vi "Find Previous File.vi"(7 "Baseline Directory":path, 8 "error in":errorcluster, 10 "Relative Path":string, 11 "Response String":string) -> (0 "error out":errorcluster, 3 "Previous Name":path)   [LabVIEW 2020, in "Peer Review.lvclass"]
uses:
  Peer Review.lvclass
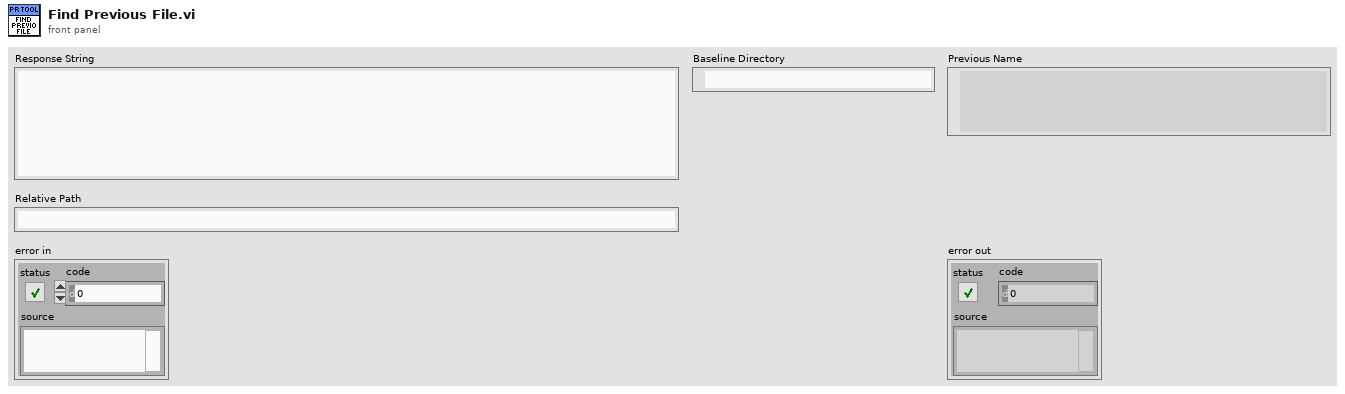
[diagram p1: front panel]
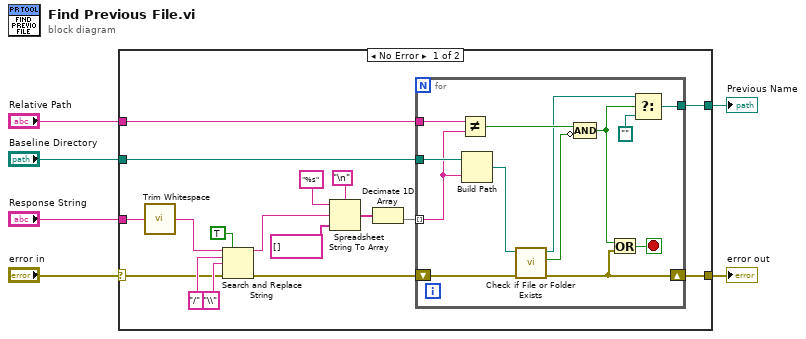
[diagram p0: block diagram]
diagram:
  n1 = case shown="No Error" "error in" {
    selector: "error in" -> [w9 w37]
    tunnel: "Baseline Directory" -> [w19 _]
    tunnel: [w17 w37] -> w5
    tunnel: [w16 _] -> w4
    tunnel: "Response String" -> [w12 _]
    tunnel: "Relative Path" -> [w7 _]
    frame No Error {
      n2 = call <vilib>:"Trim Whitespace.vi"("string"=w12) -> ("trimmed string"=w11:string)  [unwired: 1 in]
      n3 = Search and Replace String(replace all?=TRUE ("replace all? (F)"), input string=w11, search string="/", replace string="\\" ("replace string (\"\")"), error in=w9) -> (result string=w10:string, error out=w8:errorcluster)  [unwired: 3 in, 2 out]
      n4 = Spreadsheet String To Array(delimiter (Tab)="\n", format string="%s", spreadsheet string=w10, array type (2D Dbl)=string[] []) -> (array=w23:string[])
      n5 = Decimate 1D Array(w23) -> (w18:string[])  [unwired: 1 out]
      n6 = for {
        tunnel: w19 -> [w36]
        tunnel: w18 -> [w26] mode=indexing
        tunnel: w7 -> [w35]
        shift-right: [w31] -> w17
        shift-left: w8 -> [w27]
        tunnel: [w28] -> w16
        stop <- w30 stop-if-true
        n7 = Not Equal?(x=w35, y=w26) -> (x != y?=w33:bool)
        n8 = Build Path(base path=w36, name or relative path=w26) -> (appended path=w34:path)
        n9 = call <vilib>:"Check if File or Folder Exists.vi"("error in (no error)"=w27, "path"=w34) -> ("error out"=w31:errorcluster, "file or folder exists?"=w32:bool, "dup path"=w25:path)  [unwired: 7 in]
        n10 = Compound Arithmetic op=AND(w33, invert w32) -> (w29:bool)
        n11 = Or(x=w29, y=w31) -> (x .or. y?=w30:bool)
        n12 = Select(t=w25, s=w29, f=path "") -> (s? t:f=w28:path)
      }
    }
    frame Error {
    }
  }
  "error out" <- w5
  "Previous Name" <- w4
